vi "Get Auxiliary Amplifier Mode.vi"(8 "error in (no error)":errorcluster, 11 "VISA resource name":refnum<visa-resource-name>) -> (0 "error out":errorcluster, 2 "Amplifier Mode":u16, 3 "VISA resource name out":refnum<visa-resource-name>)   [LabVIEW 2014, in "Fluke 5XXX Series Multicalibrators.lvlib"]
doc: "This VI returns state of the auxiliary amplifier if the auxiliary amplifier is present in the system.\n\nNotes:\n\n(1) Instrument model 5520A and 57LFC can not use auxiliary amplifier."
uses:
  Fluke 5XXX Series Multicalibrators.lvlib
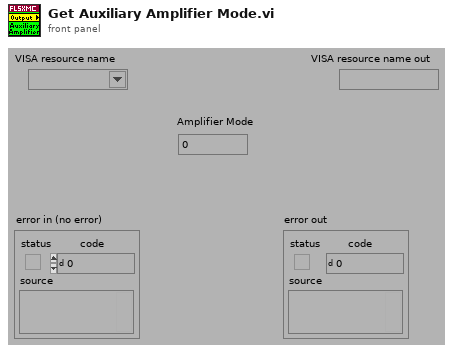
[diagram p1: front panel]
types:
  T1 = cluster{"Status":bool, "Code":i32, "Source (VI Name)":string}
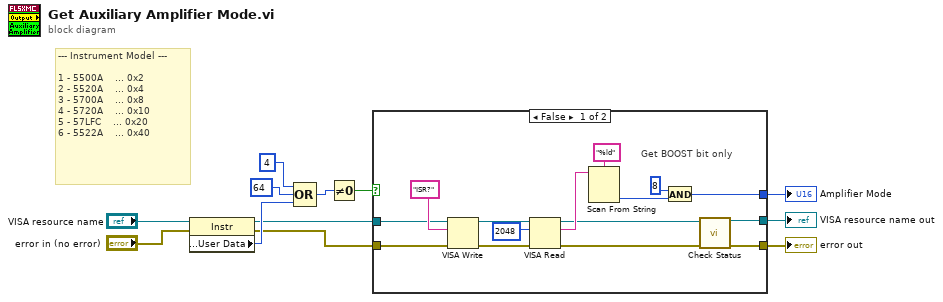
[diagram p0: block diagram]
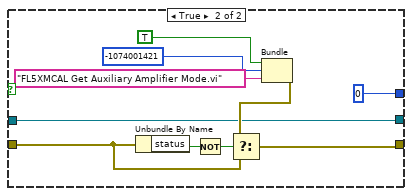
[diagram p2: hidden frame]
diagram:
  # "--- Instrument Model ---\n\n1 - 5500A    ... 0x2\n2 - 5520A    ... 0x4\n3 - 5700A    ... 0x8\n4 - 5720A    ... 0x10\n5 - 57LFC    ... 0x20\n6 - 5522A    ... 0x40"
  n1 = property class="Instr"(reference="VISA resource name", error in="error in (no error)") -> (reference out=w4:refnum<visa-resource-name>, error out=w3:errorcluster, "General Settings:User Data"=w9:u32)
  n2 = Compound Arithmetic op=OR(4 ("Numeric"), 64 ("Numeric"), w9) -> (w8:u32)
  n3 = Not Equal To 0?(x=w8) -> (x != 0?=w2:bool)
  n4 = case shown="False" w2 {
    tunnel: [w18 w28] -> w11
    tunnel: [w15 w29] -> w10
    tunnel: [w19 0] -> w12
    tunnel: w4 -> [w14 w29]
    tunnel: w3 -> [w13 w30]
    frame False {
      # "Get BOOST bit only"
      n5 = VISA Write(VISA resource name=w14, write buffer="ISR?", error in (no error)=w13) -> (VISA resource name out=w26:refnum<visa-resource-name>, error out=w25:errorcluster)  [unwired: 1 out]
      n6 = VISA Read(VISA resource name=w26, byte count=u32 2048 ("byte count (0)"), error in (no error)=w25) -> (VISA resource name out=w16:refnum<visa-resource-name>, read buffer=w22:string, error out=w17:errorcluster)  [unwired: 1 out]
      n7 = Scan From String(format string="%ld", input string=w22) -> (output 1=w20:i32)  [unwired: 3 in, 3 out]
      n8 = And(x=8, y=w20) -> (x .and. y?=w19:i32)
      n9 = call "Check Status.vi"("VISA resource name"=w16, "error in (no error)"=w17) -> ("VISA resource name out"=w15:refnum<visa-resource-name>, "error out"=w18:errorcluster)  [unwired: 12 in]
    }
    frame True {
      n10 = Unbundle By Name(w30) -> ("status"=w33:bool)
      n11 = Not(x=w33) -> (.not. x?=w32:bool)
      n12 = Bundle("Status"=TRUE, "Code"=-1074001421, "Source (VI Name)"="FL5XMCAL Get Auxiliary Amplifier Mode.vi") -> (w31:T1)  [unwired: 1 in]
      n13 = Select(t=w31, s=w32, f=w30) -> (s? t:f=w28:errorcluster)
    }
  }
  "Amplifier Mode" <- w12
  "VISA resource name out" <- w10
  "error out" <- w11
